vi "Shutdown.vi"(11 "Volcano in":refnum<class "Volcano.lvclass">) -> (3 "Volcano out":refnum<class "Volcano.lvclass">)   [LabVIEW 2021, in "d16.lvlib" / "Volcano.lvclass"]
uses:
  Volcano.lvclass
  Volcano.lvclass/Volcano.ctl
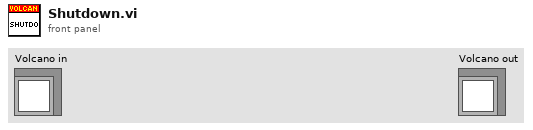
[diagram p1: front panel]
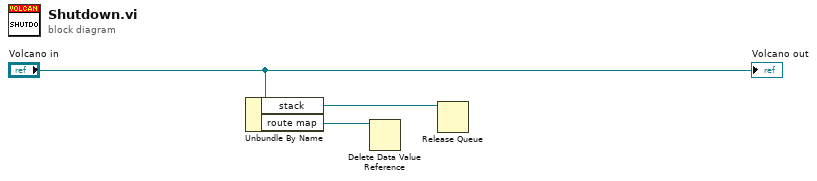
[diagram p0: block diagram]
diagram:
  n1 = Unbundle By Name("Volcano in") -> ("stack"=w2:refnum<queue>, "route map"=w1:refnum<data-value>)
  n2 = Delete Data Value Reference(data value reference=w1) -> ()  [unwired: 1 in, 2 out]
  n3 = Release Queue(queue=w2) -> ()  [unwired: 2 in, 3 out]
  "Volcano out" <- "Volcano in"
